vi "R1DOControl.vi"(8 "error constant":errorcluster, 11 "LabVIEW Web Service":refnum<class "Web Service.lvclass">) -> (0 "error (out)":errorcluster)   [LabVIEW 2016]
uses:
  <vilib>/wsapi/Web Service.lvclass
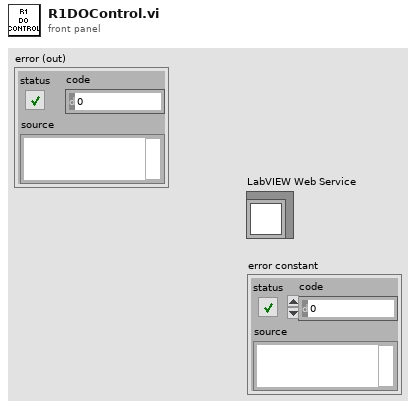
[diagram p1: front panel]
types:
  T1 = cluster{"Media Pump":bool, "Water Pump":bool, "Effluent Pump":bool, "Release Valve":bool, "Gas Pump":bool}
  T2 = cluster{"Set Point, mg/L":dbl, "Tolerance, mg/L":dbl, "N2 Valve Gain":dbl, "Air Valve Gain":dbl}
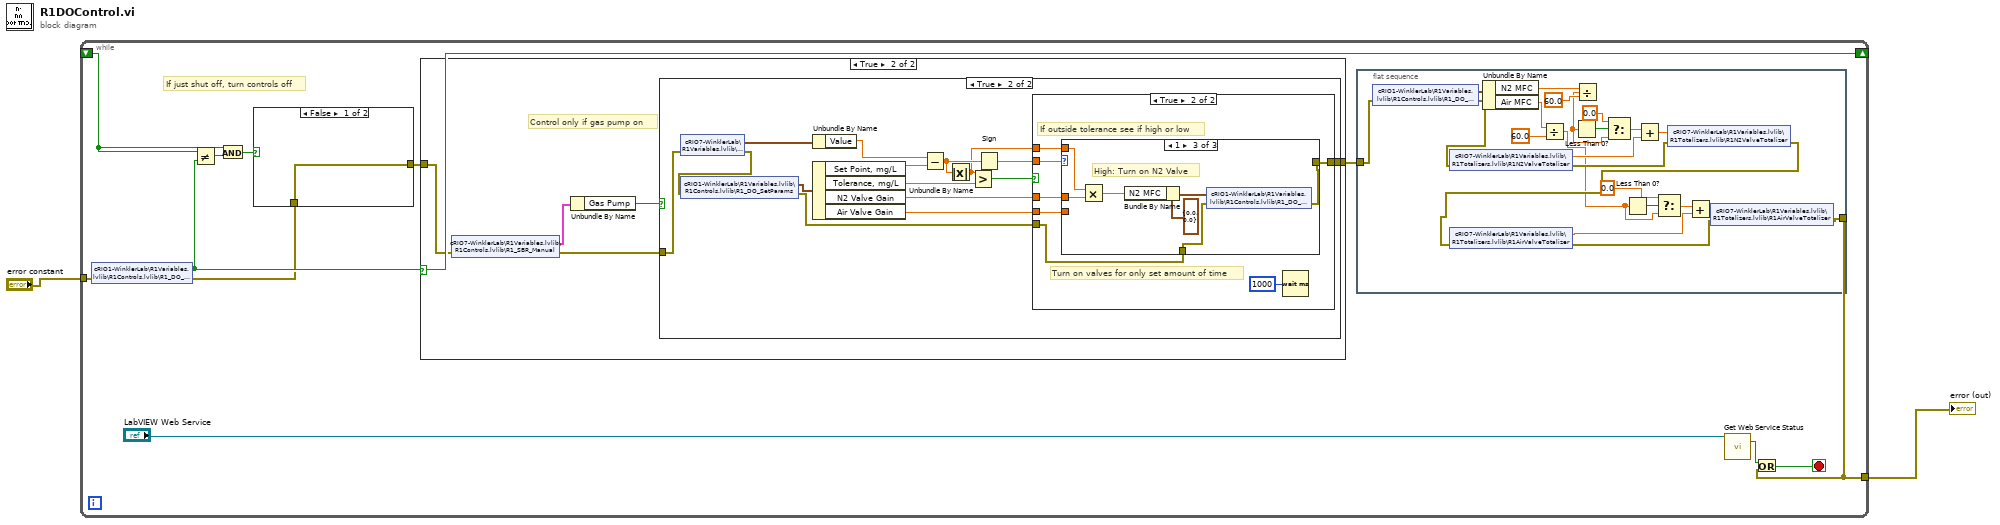
[diagram p0: block diagram]
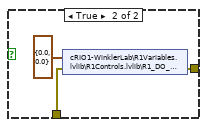
[diagram p2: hidden frame]
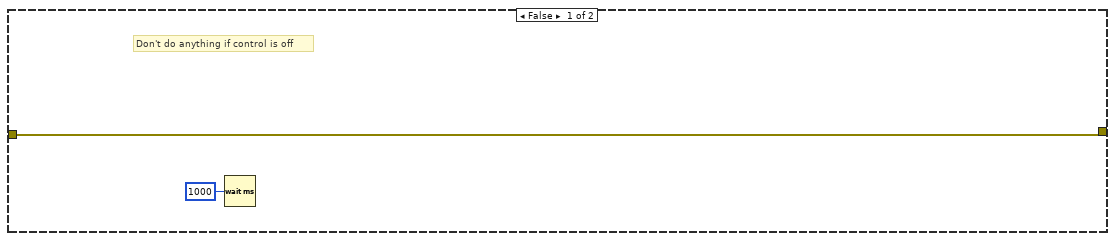
[diagram p3: hidden frame]
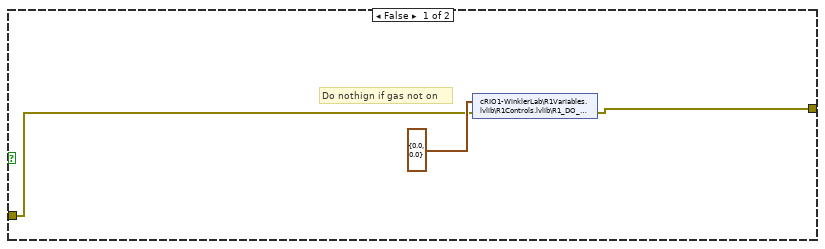
[diagram p4: hidden frame]
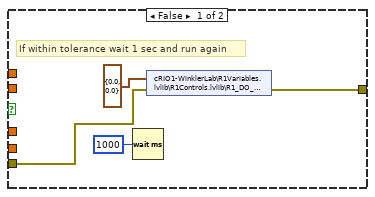
[diagram p5: hidden frame]
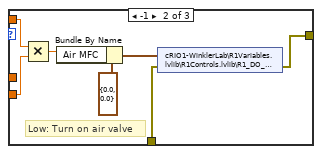
[diagram p7: hidden frame]
diagram:
  n1 = while {
    shift-right: [w10] -> _
    shift-left: _ -> [w8]
    tunnel: "error constant" -> [w7]
    tunnel: [w3] -> w1
    stop <- w12 stop-if-true
    # "If just shut off, turn controls off"
    n2 = shared-variable "cRIO1-WinklerLab\\R1Variables.lvlib\\R1Controls.lvlib\\R1_DO_Switch"(error in=w7) -> (w10:bool, error out=w6:errorcluster)
    n3 = Not Equal?(x=w8, y=w10) -> (x != y?=w9:bool)
    n4 = And(x=w8, y=w9) -> (x .and. y?=w11:bool)
    n5 = case shown="False" w11 {
      tunnel: w6 -> [w38 w40]
      tunnel: [w38 w39] -> w5
      frame False {
      }
      frame True {
        n6 = shared-variable "cRIO1-WinklerLab\\R1Variables.lvlib\\R1Controls.lvlib\\R1_DO_Manual"(cluster{"Air MFC":dbl, "N2 MFC":dbl} {"Air MFC"=0.0, "N2 MFC"=0.0} ("R1DOManual"), error in=w40) -> (error out=w39:errorcluster)
      }
    }
    n7 = case shown="True" w10 {
      tunnel: w5 -> [w42 w46]
      tunnel: [w42 w44] -> w4
      frame False {
        # "Don't do anything if control is off"
        n8 = Wait (ms)(milliseconds to wait=u32 1000) -> ()  [unwired: 1 out]
      }
      frame True {
        # "Control only if gas pump on"
        n9 = shared-variable "cRIO7-WinklerLab\\R1Variables.lvlib\\R1Controls.lvlib\\R1_SBR_Manual"(error in=w46) -> (w47:T1, error out=w45:errorcluster)
        n10 = Unbundle By Name(w47) -> ("Gas Pump"=w48:bool)
        n11 = case shown="True" w48 {
          tunnel: w45 -> [w50 w55]
          tunnel: [w49 w52] -> w44
          frame False {
            # "Do nothign if gas not on"
            n12 = shared-variable "cRIO1-WinklerLab\\R1Variables.lvlib\\R1Controls.lvlib\\R1_DO_Manual"(cluster{"Air MFC":dbl, "N2 MFC":dbl} {"Air MFC"=0.0, "N2 MFC"=0.0} ("R1DOManual"), error in=w50) -> (error out=w49:errorcluster)
          }
          frame True {
            n13 = shared-variable "cRIO7-WinklerLab\\R1Variables.lvlib\\R1Signals.lvlib\\R1DO"(error in=w55) -> (w60:cluster{"Signal":dbl, "Value":dbl}, error out=w54:errorcluster)
            n14 = shared-variable "cRIO1-WinklerLab\\R1Variables.lvlib\\R1Controls.lvlib\\R1_DO_SetParams"(error in=w54) -> (w59:T2, error out=w53:errorcluster)
            n15 = Unbundle By Name(w60) -> ("Value"=w66:dbl)
            n16 = Unbundle By Name(w59) -> ("Set Point, mg/L"=w65:dbl, "Tolerance, mg/L"=w64:dbl, "N2 Valve Gain"=w61:dbl, "Air Valve Gain"=w58:dbl)
            n17 = Subtract(x=w66, y=w65) -> (x-y=w57:dbl)
            n18 = Absolute Value(x=w57) -> (abs(x)=w56:dbl)
            n19 = Greater?(x=w56, y=w64) -> (0:w63:bool)
            n20 = Sign(1:w57) -> (0:w62:dbl)
            n21 = case shown="True" w63 {
              tunnel: w62 -> [_ w77]
              tunnel: w61 -> [_ w76]
              tunnel: w58 -> [_ w75]
              tunnel: w56 -> [_ w74]
              tunnel: w53 -> [w68 w72]
              tunnel: [w67 w71] -> w52
              frame False {
                # "If within tolerance wait 1 sec and run again"
                n22 = Wait (ms)(milliseconds to wait=u32 1000) -> ()  [unwired: 1 out]
                n23 = shared-variable "cRIO1-WinklerLab\\R1Variables.lvlib\\R1Controls.lvlib\\R1_DO_Manual"(cluster{"Air MFC":dbl, "N2 MFC":dbl} {"Air MFC"=0.0, "N2 MFC"=0.0} ("R1DOManual"), error in=w68) -> (error out=w67:errorcluster)
              }
              frame True {
                # "Turn on valves for only set amount of time"
                # "If outside tolerance see if high or low"
                n24 = case shown="1" w77 {
                  tunnel: w75 -> [_ w82 _]
                  tunnel: w76 -> [_ _ w90]
                  tunnel: w74 -> [_ w83 w91]
                  tunnel: w72 -> [w78 w80 w87]
                  tunnel: [w78 w79 w86] -> w71
                  frame 0, Default {
                    # "Unless tolerance is 0 this code\nshouldn't be accesible"
                  }
                  frame -1 {
                    # "Low: Turn on air valve"
                    n25 = Multiply(x=w83, y=w82) -> (x*y=w84:dbl)
                    n26 = Bundle By Name(cluster=cluster{"Air MFC":dbl, "N2 MFC":dbl} {"Air MFC"=0.0, "N2 MFC"=0.0} ("R1DOManual"), "Air MFC"=w84) -> (w81:cluster{"Air MFC":dbl, "N2 MFC":dbl})
                    n27 = shared-variable "cRIO1-WinklerLab\\R1Variables.lvlib\\R1Controls.lvlib\\R1_DO_Manual"(w81, error in=w80) -> (error out=w79:errorcluster)
                  }
                  frame 1 {
                    # "High: Turn on N2 Valve"
                    n28 = Multiply(x=w91, y=w90) -> (x*y=w89:dbl)
                    n29 = Bundle By Name(cluster=cluster{"Air MFC":dbl, "N2 MFC":dbl} {"Air MFC"=0.0, "N2 MFC"=0.0} ("R1DOManual"), "N2 MFC"=w89) -> (w88:cluster{"Air MFC":dbl, "N2 MFC":dbl})
                    n30 = shared-variable "cRIO1-WinklerLab\\R1Variables.lvlib\\R1Controls.lvlib\\R1_DO_Manual"(w88, error in=w87) -> (error out=w86:errorcluster)
                  }
                }
                n31 = Wait (ms)(milliseconds to wait=u32 1000) -> ()  [unwired: 1 out]
              }
            }
          }
        }
      }
    }
    n32 = flat-sequence {
      tunnel: w4 -> [w27]
      tunnel: [w21] -> w3
      frame #0 {
        n33 = shared-variable "cRIO1-WinklerLab\\R1Variables.lvlib\\R1Controls.lvlib\\R1_DO_Manual"(error in=w27) -> (w26:cluster{"Air MFC":dbl, "N2 MFC":dbl}, error out=w25:errorcluster)
        n34 = shared-variable "cRIO7-WinklerLab\\R1Variables.lvlib\\R1Totalizers.lvlib\\R1N2ValveTotalizer"(error in=w25) -> (w35:dbl, error out=w28:errorcluster)
        n35 = Unbundle By Name(w26) -> ("N2 MFC"=w16:dbl, "Air MFC"=w19:dbl)
        n36 = Divide(x=w19, y=60.0) -> (x/y=w18:dbl)
        n37 = Divide(x=w16, y=60.0) -> (x/y=w15:dbl)
        n38 = Less Than 0?(x=w15) -> (x < 0?=w37:bool)
        n39 = Select(t=0.0, s=w37, f=w15) -> (s? t:f=w34:dbl)
        n40 = Less Than 0?(x=w18) -> (x < 0?=w32:bool)
        n41 = Add(x=w34, y=w35) -> (x+y=w33:dbl)
        n42 = Select(t=0.0, s=w32, f=w18) -> (s? t:f=w31:dbl)
        n43 = shared-variable "cRIO7-WinklerLab\\R1Variables.lvlib\\R1Totalizers.lvlib\\R1N2ValveTotalizer"(w33, error in=w28) -> (error out=w24:errorcluster)
        n44 = shared-variable "cRIO7-WinklerLab\\R1Variables.lvlib\\R1Totalizers.lvlib\\R1AirValveTotalizer"(error in=w24) -> (w29:dbl, error out=w22:errorcluster)
        n45 = Add(x=w31, y=w29) -> (x+y=w23:dbl)
        n46 = shared-variable "cRIO7-WinklerLab\\R1Variables.lvlib\\R1Totalizers.lvlib\\R1AirValveTotalizer"(w23, error in=w22) -> (error out=w21:errorcluster)
      }
    }
    n47 = call <vilib>:"Get Web Service Status.vi"("LabVIEW Web Service"="LabVIEW Web Service") -> ("service stopping?"=w14:bool)  [unwired: 12 in, 2 out]
    n48 = Or(x=w14, y=w3) -> (x .or. y?=w12:bool)
  }
  "error (out)" <- w1
